vi "Montage I16 to U8.vi"(9 "Maximum intensity in I16 data":dbl=32767.0, 11 "I16 (positive only / 0-32767)":i16[][](array[numeric])) -> (3 "U8 (0-255)":u8[][](array[numeric]))   [LabVIEW 2020]
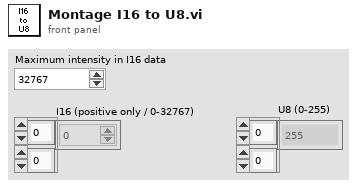
[diagram p1: front panel]
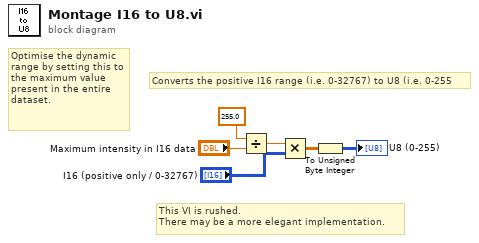
[diagram p0: block diagram]
diagram:
  # "Optimise the dynamic range by setting this to the maximum value present in the entire dataset."
  # "This VI is rushed.\nThere may be a more elegant implementation."
  # "Converts the positive I16 range (i.e. 0-32767) to U8 (i.e. 0-255"
  n1 = Divide(x=255.0 ("Numeric"), y="Maximum intensity in I16 data") -> (x/y=w5:dbl)
  n2 = Multiply(x=w5, y="I16 (positive only / 0-32767)") -> (x*y=w4:dbl[][])
  n3 = To Unsigned Byte Integer(number=w4) -> (unsigned 8bit integer=→"U8 (0-255)":u8[][])
